vi "SoundLoad.vi"(0 "Start Sound File":path) -> (1 "total number of samples/ch":u32, 2 "sound format":T1, 3 "data":waveform(dbl)[](array[waveform]), 4 "error out":errorcluster)   [LabVIEW 2013]
uses:
  <vilib>/sound2/lvsound2.llb/Sound Data Format.ctl
  <vilib>/sound2/lvsound2.llb/Sound File Read Open.vi
  <vilib>/sound2/lvsound2.llb/Sound File Info (refnum).vi
  <vilib>/sound2/lvsound2.llb/Sound File Read (DBL).vi
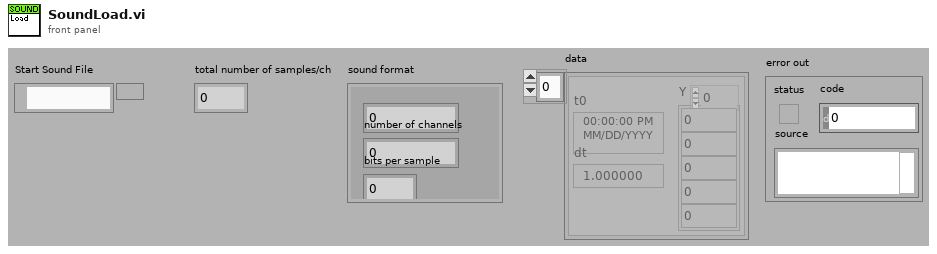
[diagram p1: front panel]
types:
  T1 = typedef "Sound Data Format.ctl" = cluster{"sample rate (S/s)":dbl, "number of channels":i32, "bits per sample":i32}
  T2 = typedef "Sound File Refnum.ctl" = refnum<file>
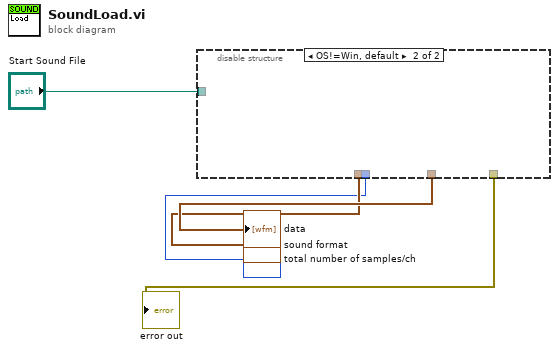
[diagram p0: block diagram]
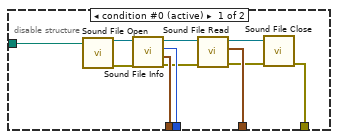
[diagram p2: hidden frame]
diagram:
  n1 = disable-structure shown="OS!=Win, default" {
    disable-tunnel: [w16 _] -> w5
    disable-tunnel: [w15 _] -> w4
    disable-tunnel: [w14 _] -> w3
    disable-tunnel: [w13 _] -> w2
    disable-tunnel: "Start Sound File" -> [w6 _]
    frame condition #0 (active) {
      n2 = call-poly <vilib>:"Sound File Open.vi"("path"=w6) -> ("error out"=w7:errorcluster, "sound file refnum"=w8:T2)  [unwired: 1 in, 8 out]
      n3 = call-poly <vilib>:"Sound File Info.vi"("error in (no error)"=w7, "sound file refnum"=w8) -> ("error out"=w10:errorcluster, "sound format"=w14:T1, "total number of samples/ch"=w13:u32, "sound file refnum out"=w9:T2)  [unwired: 6 out]
      n4 = call-poly <vilib>:"Sound File Read.vi"("error in (no error)"=w10, "sound file refnum"=w9) -> ("error out"=w12:errorcluster, "data"=w15:waveform(dbl)[], "sound file refnum out"=w11:T2)  [unwired: 3 in, 4 out]
      n5 = call <vilib>:"Sound File Close.vi"("error in (no error)"=w12, "sound file refnum"=w11) -> ("error out"=w16:errorcluster)  [unwired: 9 out]
    }
    frame condition #1 {
    }
  }
  "error out" <- w5
  "data" <- w4
  "sound format" <- w3
  "total number of samples/ch" <- w2
